vi "Send Software Trigger.vi"(8 "error in (no error)":errorcluster, 11 "VISA resource name":refnum<visa-resource-name>) -> (0 "error out":errorcluster, 3 "VISA resource name out":refnum<visa-resource-name>)   [LabVIEW 2016, in "Agilent E4980.lvlib"]
doc: "Triggers the LCR meter, then the instrument invalidates all measurement results and starts a new measuring cycle with the current settings. \n\n<B>Notes:</B>\n(1) You have to set the trigger source as Bus when sending the trigger.\n\n(2) The instrument should be in \"Wait for Trigger\" state when sending the trigger."
uses:
  <instrlib>/Agilent E4980/Agilent E4980.lvlib
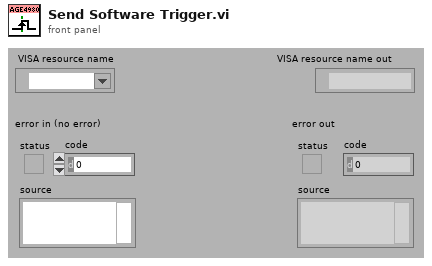
[diagram p1: front panel]
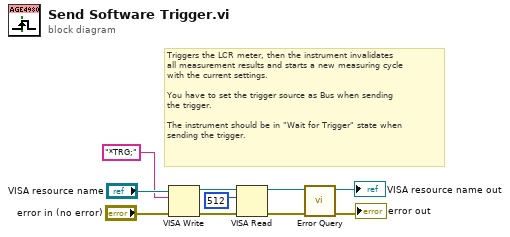
[diagram p0: block diagram]
diagram:
  # "Triggers the LCR meter, then the instrument invalidates\nall measurement results and starts a new measuring cycle\nwith the current settings.                         \n\nYou have to set the trigger source as Bus when sending\nthe trigger.\n\nThe instrument should be in \"Wait for Trigger\" state when\nsending the trigger."
  n1 = VISA Write(VISA resource name="VISA resource name", write buffer="*TRG;", error in (no error)="error in (no error)") -> (VISA resource name out=w5:refnum<visa-resource-name>, error out=w4:errorcluster)  [unwired: 1 out]
  n2 = VISA Read(VISA resource name=w5, byte count=u32 512, error in (no error)=w4) -> (VISA resource name out=w3:refnum<visa-resource-name>, error out=w2:errorcluster)  [unwired: 2 out]
  n3 = call <instrlib>:"Error Query.vi"("error in (no error)"=w2, "VISA resource name"=w3) -> ("error out"=→"error out":errorcluster, "VISA resource name out"=→"VISA resource name out":refnum<visa-resource-name>)  [unwired: 6 in, 2 out]
